vi "PFI-28000-System-Constant_Supported Cards.vi"() -> (8 "Supported Cards":string[](array[string]))   [LabVIEW 2017, in "PFI-28000-System.lvclass"]
uses:
  PFI-28000-System.lvclass
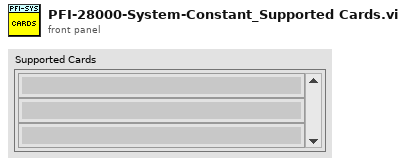
[diagram p1: front panel]
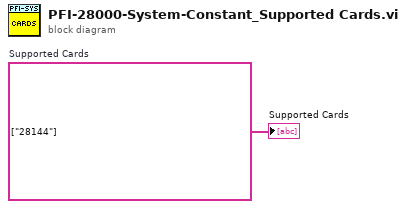
[diagram p0: block diagram]
diagram:
  w1 = string[] ["28144"]  # Supported Cards
  "Supported Cards" <- w1
